vi "OvershootCalc.vi"(0 "Motion Settings In in":T2 {"3rd Axis" items=["x", "y", "z", "w"]; "Xtra planes" min=1; "Xtra plane\ndistance  (um)" min=0; "Distance between\nscan planes (um)" format="%.2f"; "Distance between\nscan lines (um)" format="%.2f"; "SMAC Axis" items=["None"=0, "Axis 1"=1, "Axis 2"=2, "Axis 3"=3, "Axis 4"=4, "Axis 5"=5, "Axis 6"=6, "Axis 7"=7, "Axis 8"=8, "Vector Space 1"=17, "Vector Space 2"=18, "Vector Space 3"=19, "Vector Space 4"=20]; "Motion Bd ID" min=1 max=32 step=1}, 2 "Num of trigs to overshoot (2.5)":sgl=2.5, 3 "Distance between\nscan lines (um)":sgl, 4 "rmax overshoot":sgl=200.0, 5 "Total Length of Scan (mm)":sgl) -> (1 "Overshoot Count":sgl, 6 "Motion Settings out":T2 {"3rd Axis" items=["x", "y", "z", "w"]; "Xtra planes" min=1; "Xtra plane\ndistance  (um)" min=0; "Distance between\nscan planes (um)" format="%.2f"; "Distance between\nscan lines (um)" format="%.2f"; "SMAC Axis" items=["None"=0, "Axis 1"=1, "Axis 2"=2, "Axis 3"=3, "Axis 4"=4, "Axis 5"=5, "Axis 6"=6, "Axis 7"=7, "Axis 8"=8, "Vector Space 1"=17, "Vector Space 2"=18, "Vector Space 3"=19, "Vector Space 4"=20]; "Motion Bd ID" min=1 max=32 step=1}, 7 "scan pair out":T1, 8 "Steps per mm":i32)   [LabVIEW 2022 SP3]
uses:
  NI_controller/-NI_MotionRoutines/MotionParameters.ctl
  NI_controller/-NI_MotionRoutines/MotionSys.ctl
  ScanAxis.ctl
  3rdAxis.ctl
panel:
  # "1-D and 2-D B scan settings"
  # "1-D and 2-D B scan settings"
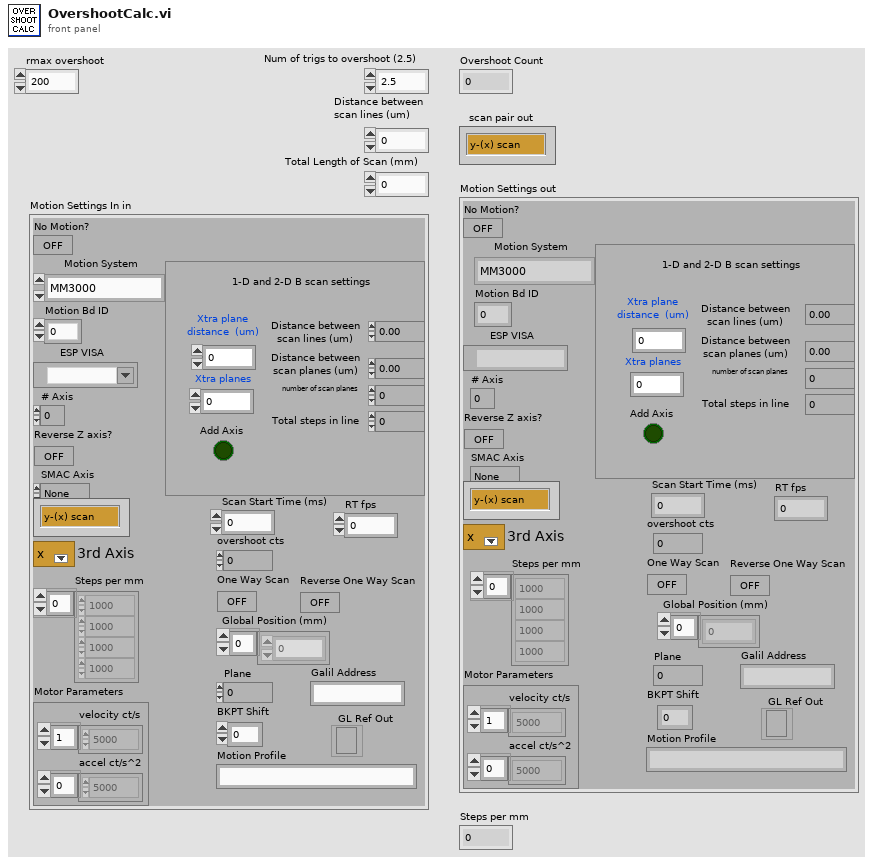
[diagram p1: front panel]
types:
  T1 = typedef "ScanAxis.ctl" = enum16{"y-(x) scan", "x-(y) scan", "z-(x) scan", "z-(y) scan", "y-(z) scan", "x-(z) scan", "w-(x) scan", "w-(y) scan", "w-(z) scan", "x-(w) scan", "y-(w) scan", "z-(w) scan"}
  T2 = typedef "MotionParameters.ctl" = cluster{"No Motion?":bool, "Motion System":T3, "Motion Bd ID":u8, "Motion Profile":string, "# Axis":i8, "Reverse Z axis?":bool, "SMAC Axis":u16, "scan pair":T1, "RT fps":sgl, "Steps per mm":i32[], "Motor Parameters":cluster{"velocity ct/s":dbl[], "accel ct/s^2":dbl[]}, "One Way Scan":bool, "Reverse One Way Scan":bool, "Global Position (mm)":dbl[], "Plane":i32, "Distance between\nscan lines (um)":sgl, "Distance between\nscan planes (um)":sgl, "number of scan planes":i32, "Total steps in line":i32, "Xtra plane\ndistance  (um)":i32, "Xtra planes ":i32, "Add Axis":bool, "overshoot cts":i32, "BKPT Shift":i32, "Scan Start Time (ms)":u32, "ESP VISA":refnum<visa-resource-name>, "3rd Axis":T4, "GL Ref Out":refnum<k7>, "Galil Address":string}
  T3 = typedef "MotionSys.ctl" = enum16{"MM3000", "NI 735x", "Newport ESP", "No Motion Card", "Galil"}
  T4 = typedef "3rdAxis.ctl" = u16
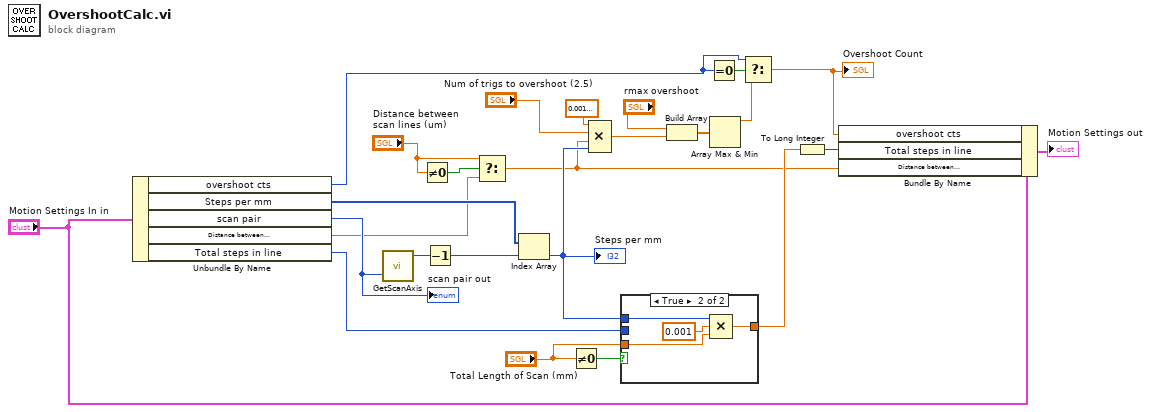
[diagram p0: block diagram]
diagram:
  n1 = Unbundle By Name("Motion Settings In in") -> ("overshoot cts"=w2:i32, "Steps per mm"=w18:i32[], "scan pair"=w16:T1, "Distance between\nscan lines (um)"=w11:sgl, "Total steps in line"=w10:i32)
  "scan pair out" <- w16
  n2 = call "GetScanAxis.vi"("scan pair"=w16) -> ("Axis 1"=w19:i32)  [unwired: 1 in, 2 out]
  n3 = Not Equal To 0?(x="Distance between\nscan lines (um)") -> (x != 0?=w12:bool)
  n4 = Decrement(x=w19) -> (x-1=w17:i32)
  n5 = Select(t="Distance between\nscan lines (um)", s=w12, f=w11) -> (s? t:f=w1:sgl)
  n6 = Index Array(array=w18, index=w17) -> (element=w15:i32)
  "Steps per mm" <- w15
  n7 = Not Equal To 0?(x="Total Length of Scan (mm)") -> (x != 0?=w9:bool)
  n8 = Compound Arithmetic op=MULTIPLY(sgl 0.001 ("value"), "Num of trigs to overshoot (2.5)", w1, w15) -> (w23:sgl)
  n9 = case shown="True" w9 {
    tunnel: w15 -> [_ w29]
    tunnel: [w26 w28] -> w14
    tunnel: "Total Length of Scan (mm)" -> [_ w27]
    tunnel: w10 -> [w26 _]
    frame False {
    }
    frame True {
      n10 = Compound Arithmetic op=MULTIPLY(w29, 0.001, w27) -> (w28:dbl)
    }
  }
  n11 = Build Array("rmax overshoot", w23) -> (w22:sgl[])
  n12 = Equal To 0?(x=w2) -> (x = 0?=w6:bool)
  n13 = Array Max & Min(array=w22) -> (max value=w5:sgl)  [unwired: 3 out]
  n14 = Select(t=w2, s=w6, f=w5) -> (s? t:f=w4:sgl)
  "Overshoot Count" <- w4
  n15 = To Long Integer(number=w14) -> (32bit integer=w7:i32)
  n16 = Bundle By Name(cluster="Motion Settings In in", "overshoot cts"=w4, "Total steps in line"=w7, "Distance between\nscan lines (um)"=w1) -> (→"Motion Settings out":T2)
